vi "Set Value of LabVIEW Array.vi"(8 "error in (no error)":errorcluster, 10 "LabVIEW Array":refnum<vi>, 11 "JSON Tree Array":variant) -> (0 "error out":errorcluster)   [LabVIEW 2013, in "i3-json.lvlib"]
doc: "This VI takes a JSON Node (all types besides JSON Object) and assigns the value to the LabVIEW Base Type of compatible reference.\n\nIf the LabVIEW base type is an array of boolean, numeric, or string this function will attempt to check if a JSON Array type will map"
uses:
  i3-json.lvlib
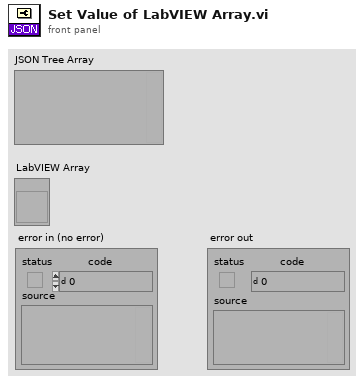
[diagram p1: front panel]
types:
  T1 = enum8{"Enabled", "Disabled", "Disabled and Grayed Out"}
  T2 = typedef "Type Enum.ctl" = enum8{"Void", "I8", "I16", "I32", "I64", "U8", "U16", "U32", "U64", "Single Float", "Double Float", "Extended Float", "Single Complex", "Double Complex", "Extended Complex", "Enum I8 NEVER", "Enum I16 NEVER", "Enum I32 NEVER", "Enum I64 NEVER", "Enum U8", "Enum U16", "Enum U32", "Enum U64", "Single Float With Unit", "Double Float With Unit", "Extended Float With Unit", "Single Complex With Unit", "Double Complex With Unit", "Extended Complex With Unit", "boolU16", "Boolean", "String", "Handle", "Path", "Picture", "C String", "Pascal String", "Tag", "SubString", "Array", "SubArray", "Cluster", "Numeric Cluster", "Variant", "LV Variant", "Measure Data (waveform)", "Refnum", "ExtData", "function", "Typedef", "Poly VI", "bad wire", "LabVIEW Class Instance"}
  T3 = typedef "i3-json.lvlib/JSON Type.ctl" = enum8{"JSON Compatible", "JSON Array", "JSON Object", "JSON Null", "Double", "String", "Boolean", "Unknown", "Data JSON string"}
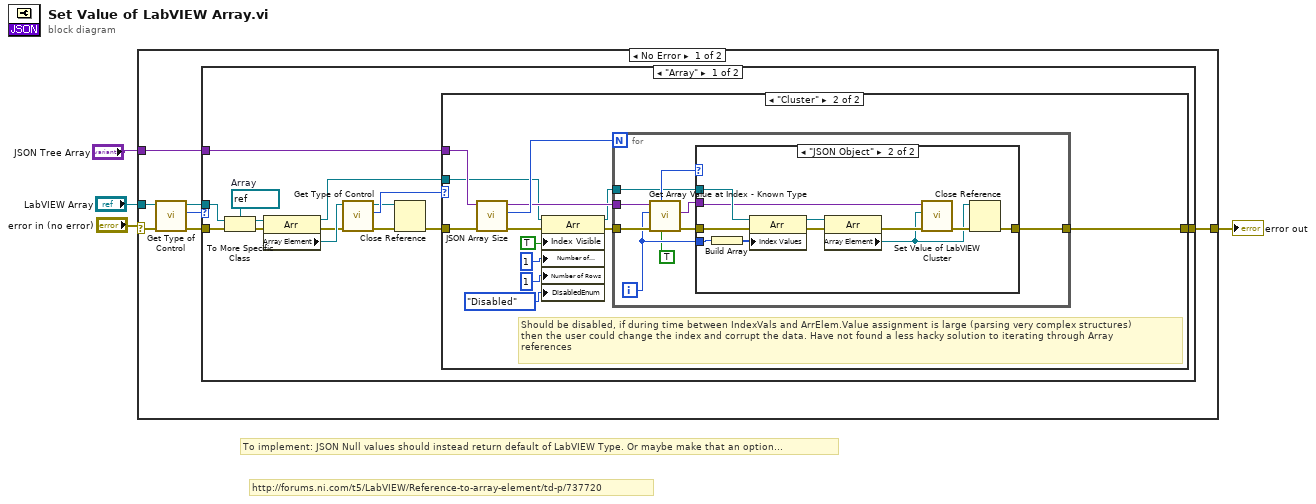
[diagram p0: block diagram]
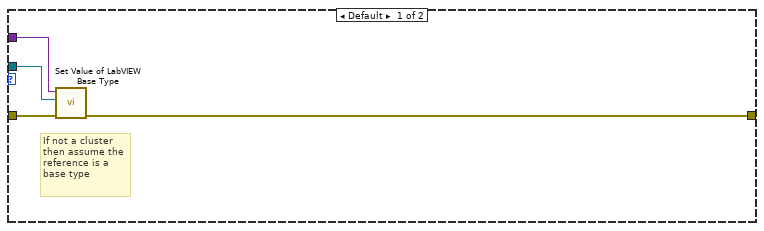
[diagram p2: hidden frame]
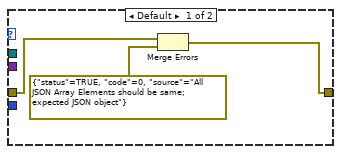
[diagram p3: hidden frame]
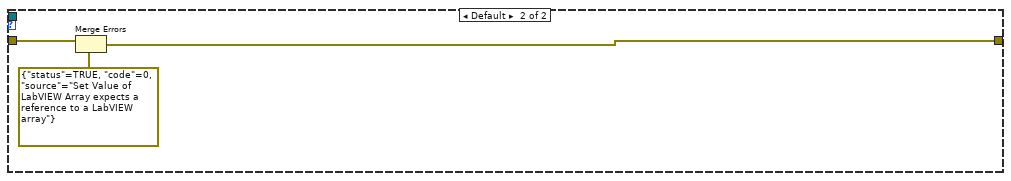
[diagram p4: hidden frame]
diagram:
  # "http://forums.ni.com/t5/LabVIEW/Reference-to-array-element/td-p/737720"
  # "To implement: JSON Null values should instead return default of LabVIEW Type. Or maybe make that an option..."
  n1 = case shown="No Error" "error in (no error)" {
    selector: "error in (no error)" -> [w11 w69]
    tunnel: "LabVIEW Array" -> [w10 _]
    tunnel: "JSON Tree Array" -> [w7 _]
    tunnel: [w5 w69] -> w1
    frame No Error {
      n2 = call <vilib>:"Get Type of Control.vi"("error in (no error)"=w11, "Control Ref In"=w10) -> ("error out"=w6:errorcluster, "Type Enum"=w9:T2, "Control Ref Out"=w8:refnum<vi>)  [unwired: 7 in]
      n3 = case shown="\"Array\"" w9 {
        tunnel: w8 -> [w24 _]
        tunnel: w7 -> [w19 _]
        tunnel: w6 -> [w25 w68]
        tunnel: [w17 w67] -> w5
        frame "Array" {
          w18 = refnum<vi> refnum  # Array
          n4 = To More Specific Class(target class=w18, reference=w24, error in=w25) -> (specific class reference=w16:refnum<vi>, error out=w23:errorcluster)
          n5 = property class="Arr"(reference=w16, error in=w23) -> (reference out=w12:refnum<vi>, error out=w21:errorcluster, "Array Element"=w22:refnum<vi>)
          n6 = call <vilib>:"Get Type of Control.vi"("error in (no error)"=w21, "Control Ref In"=w22) -> ("error out"=w15:errorcluster, "Type Enum"=w20:T2, "Control Ref Out"=w13:refnum<vi>)  [unwired: 7 in]
          n7 = Close Reference(reference=w13, error in (no error)=w15) -> (error out=w14:errorcluster)
          n8 = case shown="\"Cluster\"" w20 {
            tunnel: w14 -> [w29 w42]
            tunnel: w19 -> [w27 w41]
            tunnel: w12 -> [w28 w32]
            tunnel: [w26 w30] -> w17
            frame Default {
              # "If not a cluster then assume the reference is a base type"
              n9 = call "Set Value of LabVIEW Base Type.vi"("error in (no error)"=w29, "LabVIEW Base Type"=w28, "JSON Tree Node"=w27) -> ("error out"=w26:errorcluster)  [unwired: 8 in]
            }
            frame "Cluster" {
              # "Should be disabled, if during time between IndexVals and ArrElem.Value assignment is large (parsing very complex structures)\nthen the user could change the index and corrupt the data. Have not found a less hacky solution to iterating through Array\nreferences"
              n10 = call "JSON Array Size.vi"("error in (no error)"=w42, "JSON Tree In (JSON Array)"=w41) -> ("error out"=w34:errorcluster, "Array Size"=w40:i32, "JSON Tree Passthrough (JSON Array)"=w39:variant)  [unwired: 7 in]
              n11 = property class="Arr"(reference=w32, error in=w34, "Index Visible"=TRUE, "Number of Columns"=u32 1, "Number of Rows"=u32 1, "DisabledEnum"=T1."Disabled" ("Disabled")) -> (reference out=w31:refnum<vi>, error out=w33:errorcluster)
              n12 = for {
                N: w40 -> [_]
                tunnel: w39 -> [w50]
                tunnel: w33 -> [w51]
                tunnel: w31 -> [w45]
                tunnel: [w46] -> w30
                i -> [w44]
                n13 = call "Get Array Value at Index - Known Type.vi"("Get Value as JSON Tree? (F)"=TRUE, "error in (no error)"=w51, "Index"=w44, "JSON Tree In (JSON Array)"=w50) -> ("error out"=w48:errorcluster, "Value"=w47:variant, "JSON Type"=w49:T3)  [unwired: 2 in, 3 out]
                n14 = case shown="\"JSON Object\"" w49 {
                  tunnel: w48 -> [w53 w65]
                  tunnel: w47 -> [_ w58]
                  tunnel: [w52 w57] -> w46
                  tunnel: w45 -> [_ w62]
                  tunnel: w44 -> [_ w64]
                  frame Default {
                    n15 = Merge Errors(w53, errorcluster {"status"=TRUE, "code"=0, "source"="All JSON Array Elements should be same; expected JSON object"} ("error in")) -> (w52:errorcluster)
                  }
                  frame "JSON Object" {
                    n16 = Build Array(w64) -> (w63:i32[])
                    n17 = property class="Arr"(reference=w62, error in=w65, "Index Values"=w63) -> (reference out=w61:refnum<vi>, error out=w60:errorcluster)
                    n18 = property class="Arr"(reference=w61, error in=w60) -> (error out=w59:errorcluster, "Array Element"=w55:refnum<vi>)  [unwired: 1 out]
                    n19 = call "Set Value of LabVIEW Cluster.vi"("error in (no error)"=w59, "LabVIEW Cluster"=w55, "JSON Tree Object"=w58) -> ("error out"=w56:errorcluster)  [unwired: 8 in]
                    n20 = Close Reference(reference=w55, error in (no error)=w56) -> (error out=w57:errorcluster)
                  }
                }
              }
            }
          }
        }
        frame Default {
          n21 = Merge Errors(w68, errorcluster {"status"=TRUE, "code"=0, "source"="Set Value of LabVIEW Array expects a reference to a LabVIEW array"} ("error in")) -> (w67:errorcluster)
        }
      }
    }
    frame Error {
    }
  }
  "error out" <- w1
